vi "CMD_02_Set_DAC2.vi"(9 "Input, V":dbl min=-10.0 max=10.0, 11 "VISA resource name":refnum<visa-resource-name>) -> (3 "VISA resource name out":refnum<visa-resource-name>)   [LabVIEW 2017]
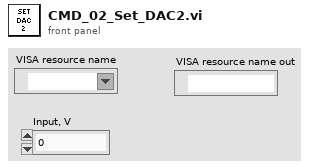
[diagram p1: front panel]
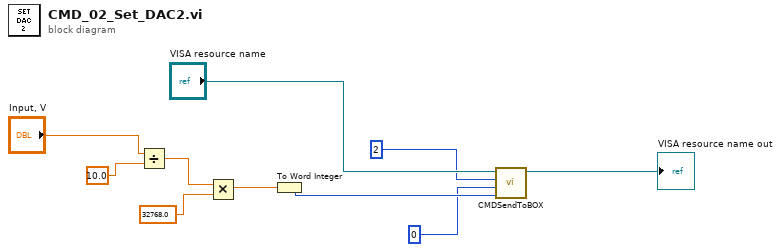
[diagram p0: block diagram]
diagram:
  n1 = Divide(x="Input, V", y=10.0) -> (x/y=w7:dbl)
  n2 = Multiply(x=w7, y=32768.0) -> (x*y=w8:dbl)
  n3 = To Word Integer(number=w8) -> (16bit integer=w2:i16)
  n4 = call "CMDSendToBOX.vi"("arg2"=w2, "arg1"=i16 0 ("arg2"), "CMD"=i8 2, "VISA resource name"="VISA resource name") -> ("VISA resource name out"=→"VISA resource name out":refnum<visa-resource-name>)  [unwired: 7 in]
